vi "PS Current.vi"() -> ()   [LabVIEW 2019]
panel:
  in  "Field [T]":dbl format="%.5f"
  out "error out":errorcluster
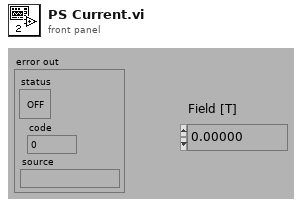
[diagram p1: front panel]
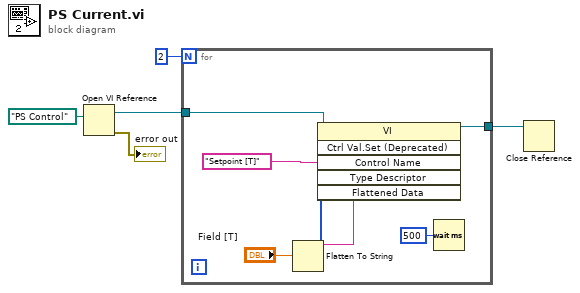
[diagram p0: block diagram]
diagram:
  n1 = Open VI Reference(vi path=path "PS Control") -> (vi reference=w1:refnum<vi>, error out=→"error out":errorcluster)  [unwired: 5 in]
  n2 = for {
    N: 2 -> [_]
    tunnel: w1 -> [w12]
    tunnel: [w7] -> w2
    n3 = Flatten To String(anything="Field [T]") -> (data string=w9:string, type string=w10:i16[])  [unwired: 3 in, 1 out]
    n4 = invoke class="VI" method="Ctrl Val.Set (Deprecated)"(reference=w12, "Control Name"="Setpoint [T]", "Type Descriptor"=w10, "Flattened Data"=w9) -> (reference out=w7:refnum<vi>)  [unwired: 2 in, 5 out]
    n5 = Wait (ms)(milliseconds to wait=u32 500) -> ()  [unwired: 1 out]
  }
  n6 = Close Reference(reference=w2) -> ()  [unwired: 1 in, 1 out]
